vi "Notify Iteration.vi"(8 "error in (no error)":errorcluster, 10 "Iterate (T)":bool=TRUE, 11 "Iterator NR Actor in":refnum<class "Iterator NR Actor.lvclass">) -> (0 "error out":errorcluster, 3 "Iterator NR Actor out":refnum<class "Iterator NR Actor.lvclass">)   [LabVIEW 2023, in "Iterator Actor.lvlib" / "Iterator NR Actor.lvclass"]
uses:
  Iterator NR Actor.lvclass
  Iterator NR Actor.lvclass/Iterator NR Actor.ctl
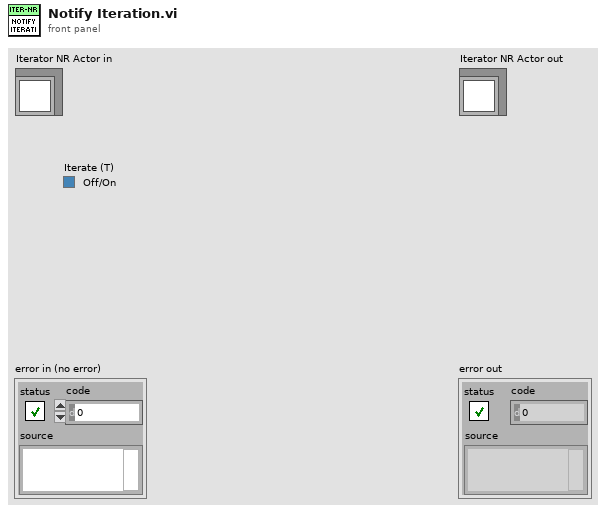
[diagram p1: front panel]
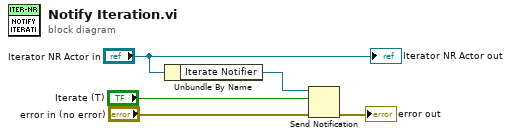
[diagram p0: block diagram]
diagram:
  n1 = Unbundle By Name("Iterator NR Actor in") -> ("Iterate Notifier"=w4:refnum<notifier>)
  n2 = Send Notification(notification="Iterate (T)", notifier=w4, error in (no error)="error in (no error)") -> (error out=→"error out":errorcluster)  [unwired: 1 out]
  "Iterator NR Actor out" <- "Iterator NR Actor in"
